vi "libssh2_sftp_stat_ex.vi"(7 "stat type":T2, 8 "error in (no error)":errorcluster, 9 "attributes in":T1, 10 "path":string, 11 "sftp":T3) -> (0 "error out":errorcluster, 1 "attributes out":T1)   [LabVIEW 2017, in "libssh2.lvlib"]
doc: "Get or set the attributes of a file or directory."
uses:
  libssh2.lvlib
  SFTP Refnum.ctl
  libssh2_sftp_attributes.ctl
  libssh2_sftp_stat_type.ctl
  Acquire Session.vi
  Release Session.vi
  Not An SFTP Refnum.vi
  <vilib>/Utility/error.llb/Error Cluster From Error Code.vi
  Global Settings.vi
  Read SFTP Refnum.vi
  Read Session Refnum.vi
  <vilib>/Utility/semaphor.llb/Acquire Semaphore.vi
  <vilib>/Utility/semaphor.llb/Release Semaphore.vi
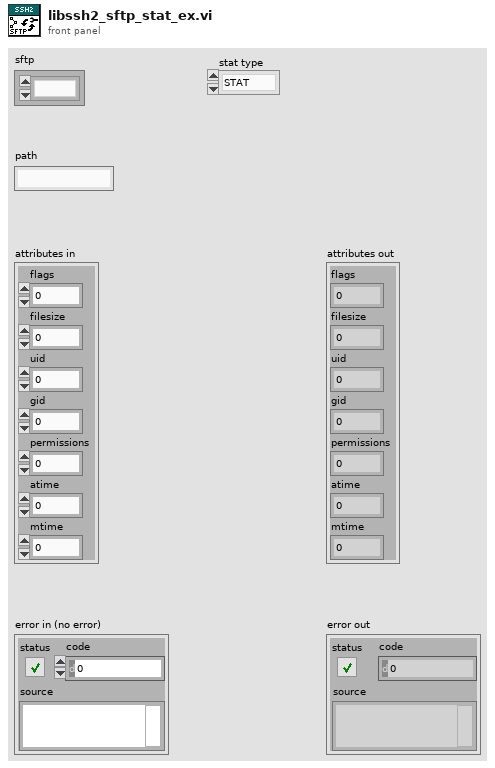
[diagram p1: front panel]
types:
  T1 = typedef "libssh2.lvlib/libssh2_sftp_attributes.ctl" = cluster{"flags":u32, "filesize":u64, "uid":u32, "gid":u32, "permissions":u32, "atime":u32, "mtime":u32}
  T2 = typedef "libssh2.lvlib/libssh2_sftp_stat_type.ctl" = enum16{"STAT", "LSTAT", "SETSTAT"}
  T3 = typedef "libssh2.lvlib/SFTP Refnum.ctl" = refnum<k1>
  T4 = cluster{"flags":u32, "<padding1>":u32, "filesize":u64, "uid":u32, "gid":u32, "permissions":u32, "atime":u32, "mtime":u32, "<padding2>":u32}
  T5 = cluster{"flags":u32, "<padding1>":u32, "filesize":u64, "uid":u32, "<padding2>":u32, "gid":u32, "<padding3>":u32, "permissions":u32, "<padding4>":u32, "atime":u32, "<padding5>":u32, "mtime":u32, "<padding6>":u32}
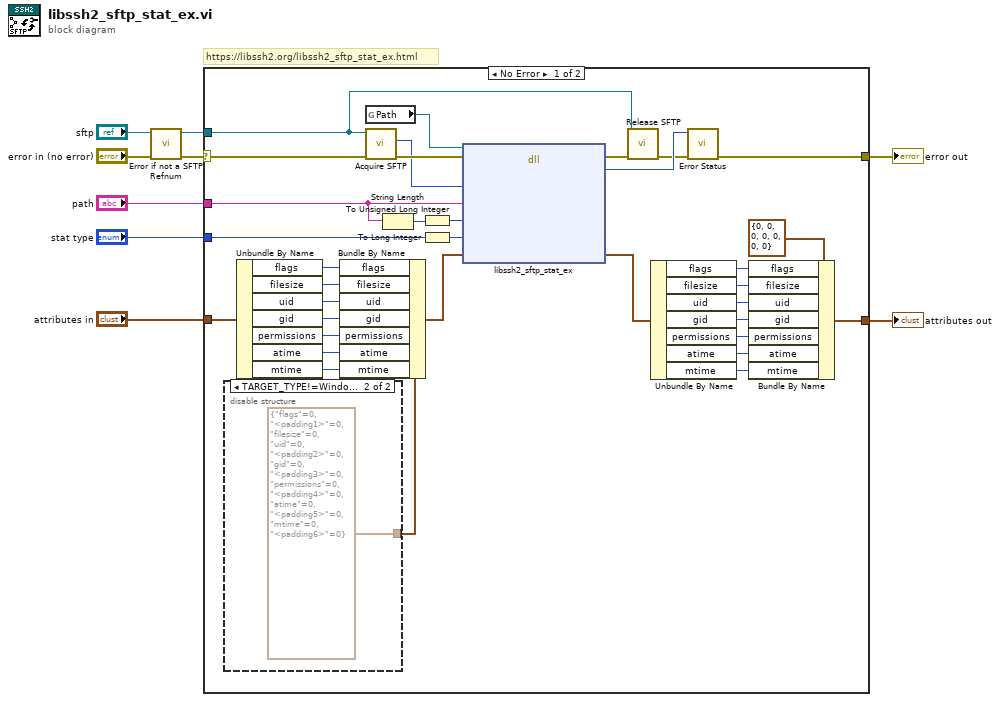
[diagram p0: block diagram]
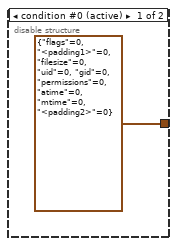
[diagram p2: hidden frame]
diagram:
  # "https://libssh2.org/libssh2_sftp_stat_ex.html"
  n1 = call "Error if not a SFTP Refnum.vi"("error in (no error)"="error in (no error)", "sftp"="sftp") -> ("error out"=w5:errorcluster, "sftp out"=w6:T3)  [unwired: 8 in]
  n2 = case shown="No Error" w5 {
    selector: w5 -> [w42 w47]
    tunnel: w6 -> [w11 _]
    tunnel: [w38 w47] -> w7
    tunnel: [w35 w46] -> w4
    tunnel: "path" -> [w25 _]
    tunnel: "stat type" -> [w23 _]
    tunnel: "attributes in" -> [w13 w46]
    frame No Error {
      n3 = disable-structure shown="TARGET_TYPE!=Windows&&TARGET_BITNESS==64" {
        disable-tunnel: [T4 {"flags"=0, "<padding1>"=0, "filesize"=0, "uid"=0, "gid"=0, "permissions"=0, "atime"=0, "mtime"=0, "<padding2>"=0} ("attrs") T5 {"flags"=0, "<padding1>"=0, "filesize"=0, "uid"=0, "<padding2>"=0, "gid"=0, "<padding3>"=0, "permissions"=0, "<padding4>"=0, "atime"=0, "<padding5>"=0, "mtime"=0, "<padding6>"=0} ("attrs")] -> w10
        frame condition #0 (active) {
        }
        frame condition #1 {
        }
      }
      n4 = Unbundle By Name(w13) -> ("flags"=w21:u32, "filesize"=w20:u64, "uid"=w19:u32, "gid"=w18:u32, "permissions"=w17:u32, "atime"=w16:u32, "mtime"=w15:u32)
      n5 = Bundle By Name(cluster=w10, "flags"=w21, "filesize"=w20, "uid"=w19, "gid"=w18, "permissions"=w17, "atime"=w16, "mtime"=w15) -> (w14:T4)
      n6 = global read "Global Settings.vi" "Path"() -> (w43:path)
      n7 = call "Acquire SFTP.vi"("error in (no error)"=w42, "sftp"=w11) -> ("error out"=w41:errorcluster, "LIBSSH2_SFTP*"=w40:u64)  [unwired: 8 in]
      n8 = String Length(string=w25) -> (length=w26:i32)
      n9 = To Unsigned Long Integer(number=w26) -> (unsigned 32bit integer=w24:u32)
      n10 = To Long Integer(number=w23) -> (32bit integer=w22:i32)
      n11 = dll-call lib="?" fn="libssh2_sftp_stat_ex"(path in=w43, error in=w41, "sftp"=w40, "path"=w25, "path_len"=w24, "stat_type"=w22, "attrs"=w14) -> (error out=w39:errorcluster, "return value"=w37:i32, "attrs"=w36:T4)  [unwired: 5 in, 1 out]
      n12 = call "Release SFTP.vi"("error in (no error)"=w39, "sftp"=w11) -> ("error out"=w12:errorcluster)  [unwired: 9 in]
      n13 = Unbundle By Name(w36) -> ("flags"=w33:u32, "filesize"=w32:u64, "uid"=w31:u32, "gid"=w30:u32, "permissions"=w29:u32, "atime"=w28:u32, "mtime"=w27:u32)
      n14 = call "Error Status.vi"("error in (no error)"=w12, "return value"=w37) -> ("error out"=w38:errorcluster)  [unwired: 8 in, 1 out]
      n15 = Bundle By Name(cluster=T1 {"flags"=0, "filesize"=0, "uid"=0, "gid"=0, "permissions"=0, "atime"=0, "mtime"=0} ("attributes"), "flags"=w33, "filesize"=w32, "uid"=w31, "gid"=w30, "permissions"=w29, "atime"=w28, "mtime"=w27) -> (w35:T1)
    }
    frame Error {
    }
  }
  "error out" <- w7
  "attributes out" <- w4
